vi "Advanced Power Measurement - Harmonics (DAQmx).vi"() -> ()   [LabVIEW 2024]
doc: "Demonstrates how to implement advanced power measurement of harmonic parameters on a three-phase electrical power system, such as measurement of harmonic distortion factor, total harmonic distortion, harmonic power, etc. Measurement of harmonic parameters is based on a resampling algorithm."
uses:
  <vilib>/addons/Electrical Power/Power Measurement/subVIs/ep_Resampled Data.ctl
  <vilib>/Utility/error.llb/DialogType.ctl
  <vilib>/DAQmx/read.llb/DAQmx Read (Analog 1D Wfm NChan NSamp).vi
  <extravilib>/ChannelInstances/Tag-bool/Read.vi
  <extravilib>/ChannelInstances/Tag-bool/Write.vi
  <extravilib>/ChannelInstances/Tag-bool/Read With Abort.vi
  <extravilib>/ChannelInstances/Tag-bool/Write With Abort.vi
  <vilib>/DAQmx/create/channels.llb/DAQmx Create Channel (AI-Voltage-Basic).vi
  <vilib>/DAQmx/create/channels.llb/DAQmx Create Channel (AI-Current-Basic).vi
  <vilib>/DAQmx/configure/timing.llb/DAQmx Timing (Sample Clock).vi
  <extravilib>/ChannelInstances/Tag-bool/Instantiate.vi
  <extravilib>/ChannelInstances/Tag-bool/EndpointRead.vi
  <extravilib>/ChannelInstances/Tag-bool/Endpoint.vi
  <vilib>/DAQmx/miscellaneous.llb/DAQmx Fill In Error Info.vi
  <resource>/objmgr/daqmx.rc
  <vilib>/addons/Electrical Power/Power Measurement/NI_EP_Power Measurement.lvlib
panel:
  in  "Display":T1(tab)
  in  "Configuration":enum32{"DAQmx", "Others"}(tab)
  in  "number of samples per channel":i32=10000
  in  "DAQmx sample rate [Hz]":dbl=50000.0 format="%0.2f"
  in  "current channels":tag="current-input/ai0:2"
  in  "maximum current value":dbl=0.002 format="%0.3f"
  in  "minimum current value":dbl=-0.002 format="%0.3f"
  in  "voltage channels":tag="voltage-input/ai0:2"
  in  "maximum voltage value":dbl=300.0 format="%0.2f"
  in  "minimum voltage value":dbl=-300.0 format="%0.2f"
  in  "frequency range [Hz]":cluster{"minimum":dbl, "maximum":dbl}={"minimum"=45.0, "maximum"=65.0}
  in  "samples per cycle":u16=192
  in  "cycles per block":u16=10
  in  "maximum harmonic  order":u16=50
  in  "distortion factor denominator":enum16{"Fundamental value", "Total value"}(ring)
  in  "filter for frequency measurement":T2={"enable filter? (T)"=TRUE, "passband edge frequency [Hz]"=65.0, "passband ripple [dB]"=0.1, "stopband edge frequency [Hz]"=85.0, "stopband attenuation [dB]"=60.0}
  out "actual DAQmx \nsample rate  [Hz]":dbl
  out "average frequency [Hz]":dbl
  out "Voltage Waveform":T3(graph)
  out "Current Waveform":T3(graph)
  out "Voltage Harmonic Spectra":T4(graph)
  out "voltage total values":dbl[](array[numeric])
  out "voltage THD [%]":dbl[](array[numeric])
  out "voltage harmonic distortion factors [%]":dbl[][](array[numeric])
  out "current THD [%]":dbl[](array[numeric])
  out "total power value":T5
  out "harmonic power values":T6(array[cluster])
  out "power values":T7(array[cluster])
  in  "stop":bool
  # "Overview: Demonstrates how to implement advanced power measurement of harmonics on a three-phase electrical power system.\nRequirements: NI-DAQmx, Electrical Power Toolkit Full Edition\nInstructions: 1. Connect the signals you want to perform advanced power measurement of harmonics to the DAQ devices.\n                        2. Configure Settings and run this VI."
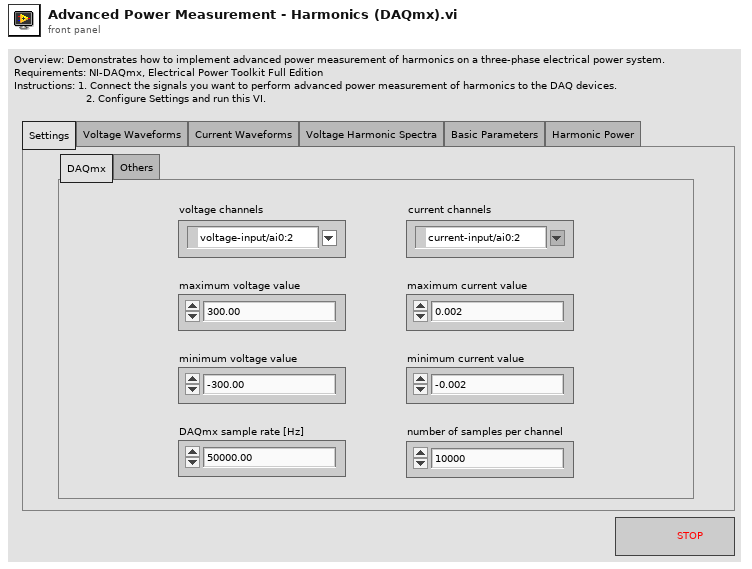
[diagram p1: front panel]
types:
  T1 = enum32{"Settings", "Voltage Waveforms", "Current Waveforms", "Voltage Harmonic Spectra", "Basic Parameters", "Harmonic Power"}
  T2 = cluster{"enable filter? (T)":bool, "passband edge frequency [Hz]":dbl, "passband ripple [dB]":dbl, "stopband edge frequency [Hz]":dbl, "stopband attenuation [dB]":dbl}
  T3 = cluster{"positions [s]":dbl[], "resampled signal":dbl[]}[]
  T4 = cluster{"order 0":dbl, "delta order":dbl, "complex spectrum":dbl[]}[]
  T5 = cluster{"active power [W]":dbl, "apparent power [VA]":dbl, "reactive power [VAR]":dbl, "power factor":dbl}
  T6 = cluster{"active power [W]":dbl, "apparent power [VA]":dbl, "reactive power [VAR]":dbl, "power factor":dbl}[][]
  T7 = cluster{"active power [W]":dbl, "apparent power [VA]":dbl, "reactive power [VAR]":dbl, "power factor":dbl}[]
  T8 = typedef "DialogType.ctl" = u16
  T9 = typedef "NI_EP_Power Measurement.lvlib/ep_Resampled Data.ctl" = cluster{"times [s]":dbl[], "resampled signal":dbl[]}
  T10 = cluster{"zero crossing times [s]":dbl[], "zero crossings per cycle":u8}
  T11 = typedef "Tag-bool.lvlib/))Channel.ctl" = refnum<queue>
  T12 = cluster{"order 0":dbl, "delta order":dbl, "complex spectrum":cdb[]}[]
  T13 = typedef "NI_EP_Basic.lvlib/basic_Power Value.ctl" = cluster{"active power [W]":dbl, "apparent power [VA]":dbl, "reactive power [VAR]":dbl, "power factor":dbl}
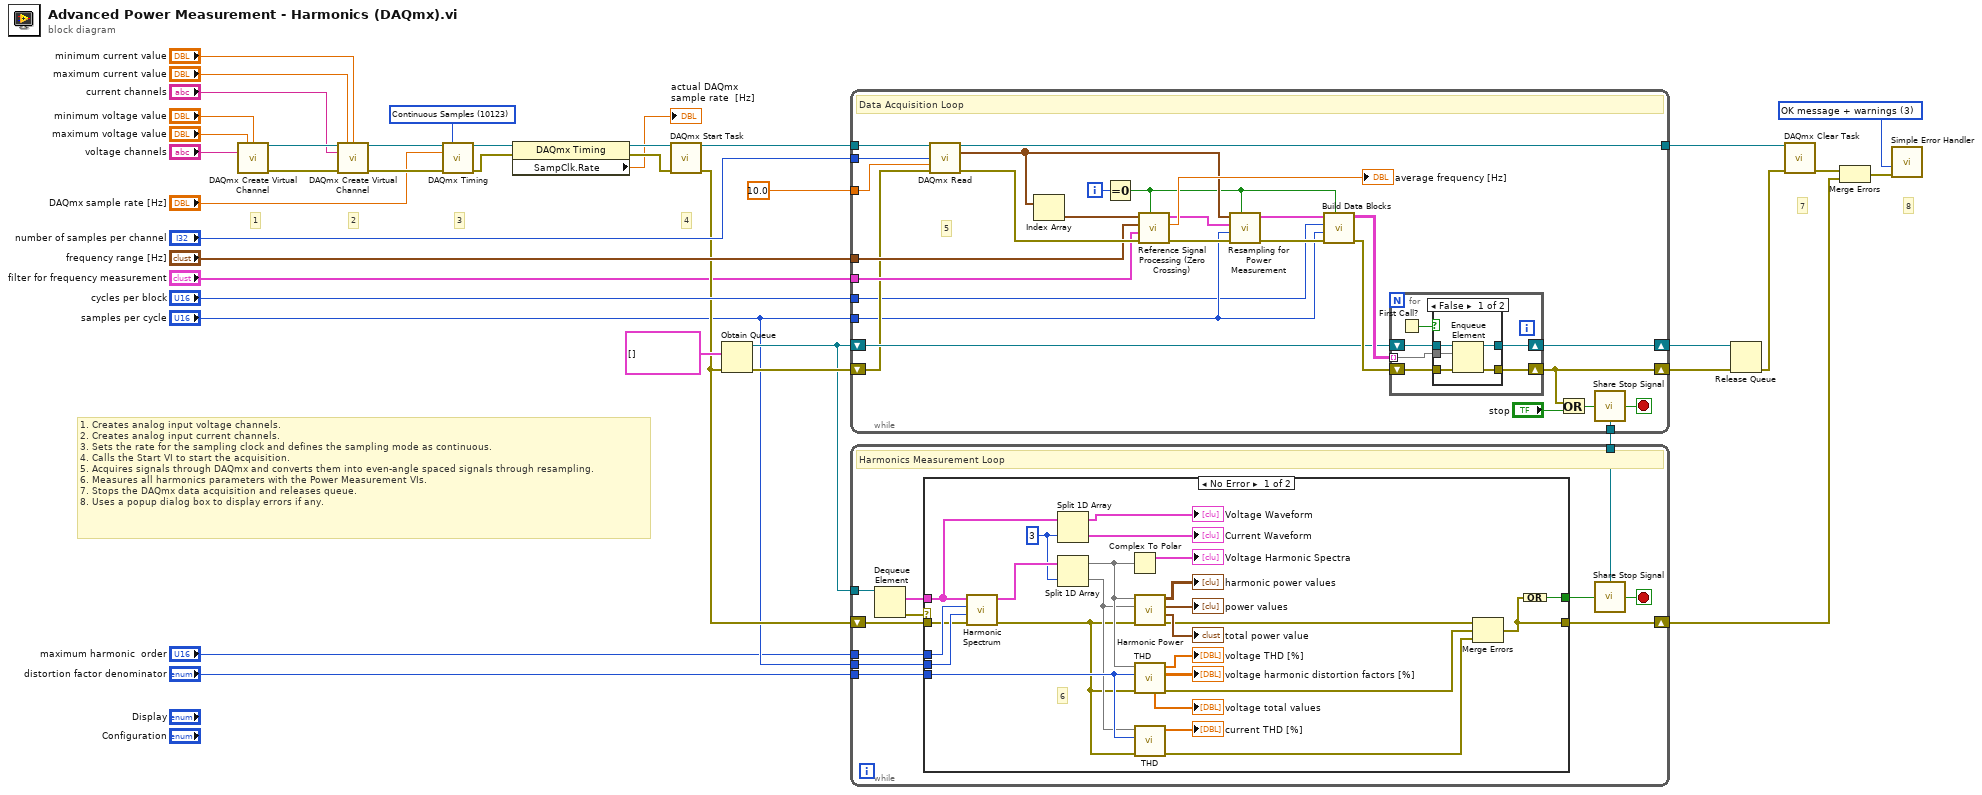
[diagram p0: block diagram]
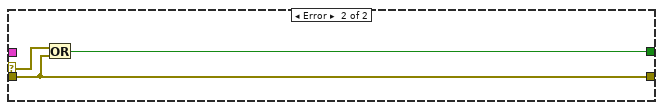
[diagram p3: hidden frame]
diagram:
  w6 = T8 3 items=["no dialog", "OK message", "continue or stop message", "OK message + warnings", "continue/stop + warnings"] ("type of dialog (OK msg:1)")
  w8 = 10123 items=["Finite Samples"=10178, "Continuous Samples"=10123, "Hardware Timed Single Point"=12522] ("sample mode")
  # "8"
  # "7"
  # "1. Creates analog input voltage channels.\n2. Creates analog input current channels.\n3. Sets the rate for the sampling clock and defines the sampling mode as continuous.\n4. Calls the Start VI to start the acquisition.\n5. Acquires signals through DAQmx and converts them into even-angle spaced signals through resampling. \n6. Measures all harmonics parameters with the Power Measurement VIs.\n7.\tStops the DAQmx data acquisition and releases queue.\n8. Uses a popup dialog box to display errors if any."
  # "4"
  # "3"
  # "2"
  # "1"
  n1 = call-poly <vilib>:"DAQmx Create Virtual Channel.vi"("maximum value"="maximum voltage value", "minimum value"="minimum voltage value", "physical channels"="voltage channels") -> ("task out"=w35:refnum<k21>, "error out"=w36:errorcluster)  [unwired: 11 in]
  n2 = call-poly <vilib>:"DAQmx Create Virtual Channel.vi"("task in"=w35, "maximum value"="maximum current value", "minimum value"="minimum current value", "physical channels"="current channels", "error in"=w36) -> ("task out"=w30:refnum<k21>, "error out"=w31:errorcluster)  [unwired: 9 in]
  n3 = call-poly <vilib>:"DAQmx Timing.vi"("task/channels in"=w30, "sample mode"=w8, "rate"="DAQmx sample rate [Hz]", "error in"=w31) -> ("task out"=w24:refnum<k21>, "error out"=w28:errorcluster)  [unwired: 10 in]
  n4 = property class="DAQmx Timing"(reference=w24, error in=w28) -> (reference out=w27:refnum<k21>, error out=w26:errorcluster, "SampClk.Rate"=→"actual DAQmx \nsample rate  [Hz]":dbl)
  n5 = call <vilib>:"DAQmx Start Task.vi"("task/channels in"=w27, "error in"=w26) -> ("task out"=w25:refnum<k21>, "error out"=w14:errorcluster)  [unwired: 12 in]
  n6 = Obtain Queue(element data type=T9[] [] ("resampled data"), error in (no error)=w14) -> (queue out=w15:refnum<queue>, error out=w19:errorcluster)  [unwired: 3 in, 1 out]
  n7 = while {
    tunnel: "number of samples per channel" -> [w66]
    tunnel: w25 -> [w67]
    tunnel: [w65] -> w21
    tunnel: "frequency range [Hz]" -> [w61]
    tunnel: "filter for frequency measurement" -> [w60]
    shift-right: [w48] -> w17
    shift-left: w15 -> [w50]
    shift-right: [w44] -> w3
    shift-left: w19 -> [w49]
    tunnel: "samples per cycle" -> [w47]
    tunnel: "cycles per block" -> [w46]
    tunnel: [w41] -> w5
    tunnel: 10.0 ("timeout") -> [w40]
    i -> [w63]
    stop <- w42 stop-if-true
    # "5"
    # "Data Acquisition Loop"
    n8 = call-poly <vilib>:"DAQmx Read.vi"("task/channels in"=w67, "number of samples per channel"=w66, "timeout"=w40, "error in"=w49) -> ("task out"=w65:refnum<k21>, "data"=w56:waveform(dbl)[], "error out"=w64:errorcluster)  [unwired: 9 in]
    n9 = Index Array(array=w56) -> (element=w62:waveform(dbl))  [unwired: 1 in]
    n10 = Equal To 0?(x=w63) -> (x = 0?=w53:bool)
    n11 = call <vilib>:"Reference Signal Processing (Zero Crossing).vi"("reset? (F)"=w53, "error in (no error)"=w64, "filter for frequency measurement"=w60, "frequency range [Hz]"=w61, "reference signal"=w62) -> ("error out"=w58:errorcluster, "average frequency [Hz]"=→"average frequency [Hz]":dbl, "zero crossing information"=w57:T10)  [unwired: 3 in, 1 out]
    n12 = call <vilib>:"Resampling for Power Measurement.vi"("reset? (F)"=w53, "error in (no error)"=w58, "samples per cycle (192)"=w47, "trigger information"=w57, "data in"=w56) -> ("error out"=w55:errorcluster, "resampled data"=w54:T9[])  [unwired: 5 in]
    n13 = call <vilib>:"Build Data Blocks.vi"("reset? (F)"=w53, "error in (no error)"=w55, "samples per cycle (192)"=w47, "cycles per block (10)"=w46, "resampled data"=w54) -> ("error out"=w52:errorcluster, "data blocks"=w51:T9[][])  [unwired: 5 in]
    n14 = for {
      shift-right: [w71] -> w48
      shift-left: w50 -> [w72]
      shift-right: [w73] -> w44
      shift-left: w52 -> [w70]
      tunnel: w51 -> [w69] mode=indexing
      n15 = First Call?() -> (First Call?: T/F=w68:bool)
      n16 = case shown="False" w68 {
        tunnel: [w78 w79] -> w73
        tunnel: w72 -> [w77 w80]
        tunnel: [w76 w80] -> w71
        tunnel: w70 -> [w75 w79]
        tunnel: w69 -> [w74 _]
        frame False {
          n17 = Enqueue Element(queue=w77, element=w74, error in (no error)=w75) -> (queue out=w76:refnum<queue>, error out=w78:errorcluster)  [unwired: 1 in, 1 out]
        }
        frame True {
        }
      }
    }
    n18 = Or(x=w44, y="stop") -> (x .or. y?=w43:bool)
    n19 = call <vilib>:"Share Stop Signal.vi"("set stop (F)"=w43) -> ("channel"=w41:T11, "stop"=w42:bool)
  }
  n20 = while {
    shift-right: [w83] -> w10
    shift-left: w14 -> [w86]
    tunnel: w15 -> [w91]
    tunnel: "samples per cycle" -> [w89]
    tunnel: "maximum harmonic  order" -> [w88]
    tunnel: "distortion factor denominator" -> [w87]
    tunnel: w5 -> [w81]
    stop <- w84 stop-if-true
    # "Harmonics Measurement Loop"
    n21 = Dequeue Element(queue=w91) -> (element=w90:T9[], error out=w85:errorcluster)  [unwired: 2 in, 2 out]
    n22 = case shown="No Error" w85 {
      selector: w85 -> [_ w119]
      tunnel: w90 -> [w97 _]
      tunnel: w89 -> [w114 _]
      tunnel: w88 -> [w113 _]
      tunnel: w86 -> [w112 w118]
      tunnel: [w100 w118] -> w83
      tunnel: w87 -> [w109 _]
      tunnel: [w93 w117] -> w82
      frame No Error {
        w92 = 3 ("index")
        # "6"
        n23 = call <vilib>:"Harmonic Spectrum.vi"("error in (no error)"=w112, "samples per cycle (192)"=w114, "maximum harmonic order (50)"=w113, "resampled data"=w97) -> ("error out"=w94:errorcluster, "harmonic spectra"=w111:T12)  [unwired: 6 in]
        n24 = Split 1D Array(array=w97, index=w92) -> (first subarray=→"Voltage Waveform":T9[], second subarray=→"Current Waveform":T9[])
        n25 = Split 1D Array(array=w111, index=w92) -> (first subarray=w110:T12, second subarray=w107:T12)
        n26 = Complex To Polar(r * e^(i*theta)=w110) -> (r=→"Voltage Harmonic Spectra":T4)  [unwired: 1 out]
        n27 = call <vilib>:"Harmonic Power.vi"("error in (no error)"=w94, "current spectra"=w107, "voltage spectra"=w110) -> ("error out"=w101:errorcluster, "total power value"=→"total power value":T13, "power values"=→"power values":T13[], "harmonic power values"=→"harmonic power values":T13[][])  [unwired: 5 in]
        n28 = call <vilib>:"THD.vi"("error in (no error)"=w94, "distortion factor denominator"=w109, "harmonic spectra"=w110) -> ("error out"=w95:errorcluster, "harmonic distortion factors [%]"=→"voltage harmonic distortion factors [%]":dbl[][], "THD [%]"=→"voltage THD [%]":dbl[], "total values"=→"voltage total values":dbl[])  [unwired: 5 in]
        n29 = call <vilib>:"THD.vi"("error in (no error)"=w94, "distortion factor denominator"=w109, "harmonic spectra"=w107) -> ("error out"=w99:errorcluster, "THD [%]"=→"current THD [%]":dbl[])  [unwired: 5 in, 2 out]
        n30 = Merge Errors(w101, w95, w99) -> (w100:errorcluster)
        n31 = Compound Arithmetic op=OR(w100) -> (w93:bool)
      }
      frame Error {
        n32 = Or(x=w119, y=w118) -> (x .or. y?=w117:bool)
      }
    }
    n33 = call <vilib>:"Share Stop Signal.vi"("set stop (F)"=w82, "channel"=w81) -> ("stop"=w84:bool)
  }
  n34 = Release Queue(queue=w17, error in (no error)=w3) -> (error out=w2:errorcluster)  [unwired: 1 in, 2 out]
  n35 = call <vilib>:"DAQmx Clear Task.vi"("task in"=w21, "error in"=w2) -> ("error out"=w1:errorcluster)  [unwired: 13 in]
  n36 = Merge Errors(w1, w10) -> (w9:errorcluster)
  n37 = call <vilib>:"Simple Error Handler.vi"("type of dialog (OK msg:1)"=w6, "error in (no error)"=w9) -> ()  [unwired: 3 in, 5 out]
